vi "Write to TCP.vi"(8 "error in":errorcluster, 11 "lia interface in":refnum<class "LIA Host Interface RT.lvclass">) -> (0 "error out":errorcluster, 3 "lia interface out":refnum<class "LIA Host Interface RT.lvclass">)   [LabVIEW 2017, in "LIA Host Interface RT.lvclass"]
uses:
  LIA Host Interface RT.lvclass
  Properties/TcpConnection_GET.vi
  Properties/OutgoingQueue_GET.vi
  shared/Lock-In Amplifier Example Shared.lvlib
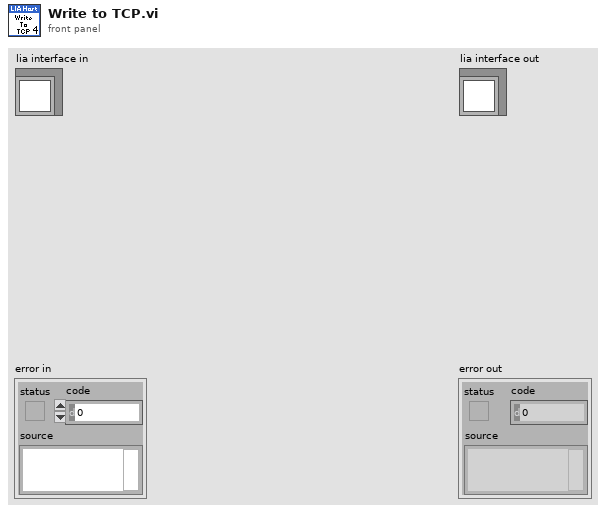
[diagram p1: front panel]
types:
  T1 = typedef "Lock-In Amplifier Example Shared.lvlib/message.ctl" = cluster{"command":u32, "payload":string}
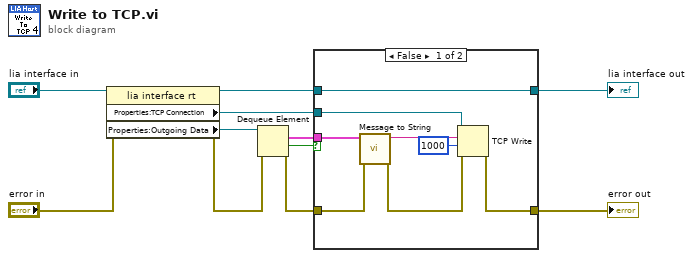
[diagram p0: block diagram]
diagram:
  n1 = property class="lia interface rt"(reference="lia interface in", error in="error in") -> (reference out=w1:refnum<class "LIA Host Interface RT.lvclass">, error out=w7:errorcluster, "Properties:TCP Connection"=w5:refnum<k5>, "Properties:Outgoing Data"=w10:refnum<queue>)
  n2 = Dequeue Element(queue=w10, error in (no error)=w7) -> (element=w9:T1, timed out?=w3:bool, error out=w6:errorcluster)  [unwired: 1 in, 1 out]
  n3 = case shown="False" w3 {
    tunnel: w9 -> [w19 _]
    tunnel: w6 -> [w18 w21]
    tunnel: w5 -> [w16 _]
    tunnel: [w13 w21] -> w4
    tunnel: [w12 w20] -> w2
    tunnel: w1 -> [w12 w20]
    frame False {
      n4 = call "Message to String.vi"("error in"=w18, "message in"=w19) -> ("error out"=w14:errorcluster, "string out"=w17:string)  [unwired: 8 in]
      n5 = TCP Write(connection ID=w16, data in=w17, error in (no error)=w14, 9:1000 ("timeout ms (25000)")) -> (error out=w13:errorcluster)  [unwired: 2 out]
    }
    frame True {
    }
  }
  "error out" <- w4
  "lia interface out" <- w2
